vi "Rajout_tiret_pourSN.vi"(11 "SN_Entrant":string="ASAC4007") -> (3 "SN: avec -":string)   [LabVIEW 2020]
panel:
  out "sous-chaîne suivante":string
  out "sous-chaîne correspondante":string
  out "sous-chaîne précédente":string
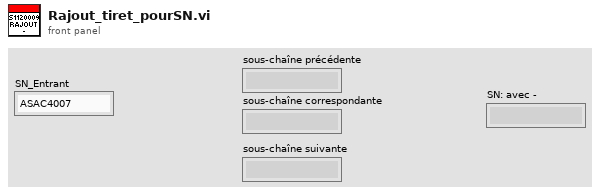
[diagram p1: front panel]
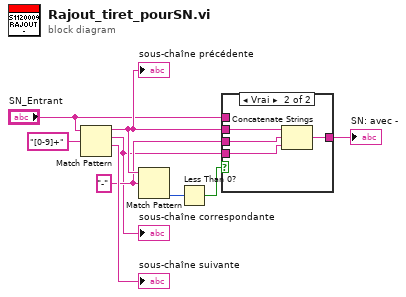
[diagram p0: block diagram]
diagram:
  w4 = "-" ("expression régulière")
  n1 = Match Pattern(string="SN_Entrant", regular expression="[0-9]+" ("chaîne/car. recherché (-)")) -> (before substring=w5:string, match substring=w3:string, after substring=→"sous-chaîne suivante":string)  [unwired: 1 in, 1 out]
  "sous-chaîne précédente" <- w5
  "sous-chaîne correspondante" <- w3
  n2 = Match Pattern(string=w5, regular expression=w4) -> (offset past match=w7:i32)  [unwired: 1 in, 3 out]
  n3 = Less Than 0?(x=w7) -> (x < 0?=w6:bool)
  n4 = case shown="Vrai" w6 {
    tunnel: w5 -> [_ w14]
    tunnel: w4 -> [_ w13]
    tunnel: w3 -> [_ w12]
    tunnel: [w10 w11] -> w2
    tunnel: "SN_Entrant" -> [w10 _]
    frame False {
    }
    frame True {
      n5 = Concatenate Strings(w14, w13, w12) -> (w11:string)
    }
  }
  "SN: avec -" <- w2
